vi "RTS Latest TDMS Data.vi"(6 "Number of values in file":u64, 8 "error in (no error)":errorcluster, 9 "Group":string, 10 "Channel":string, 11 "Refnum in":refnum<k34>) -> (0 "error out":errorcluster, 2 "Latest Data":dbl[](array[numeric]), 3 "Refnum out":refnum<k34>)   [LabVIEW 2016]
panel:
  in  "Read Times":i32=5
  out "number of buffers available":u32
  out "all buffers full?":bool
  out "read process finished?":bool
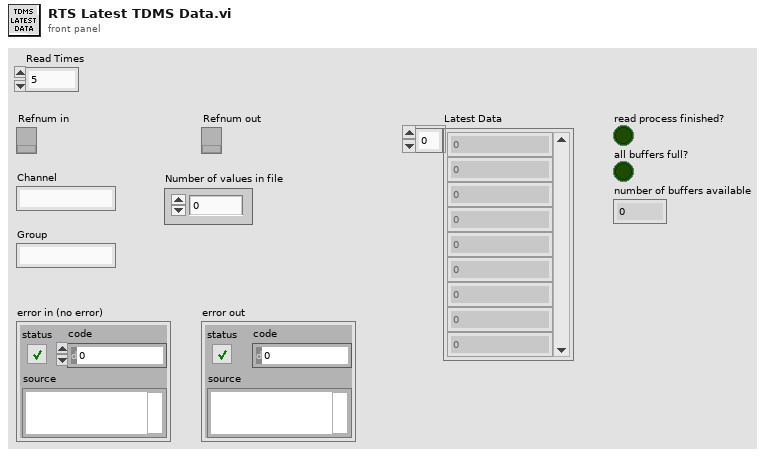
[diagram p1: front panel]
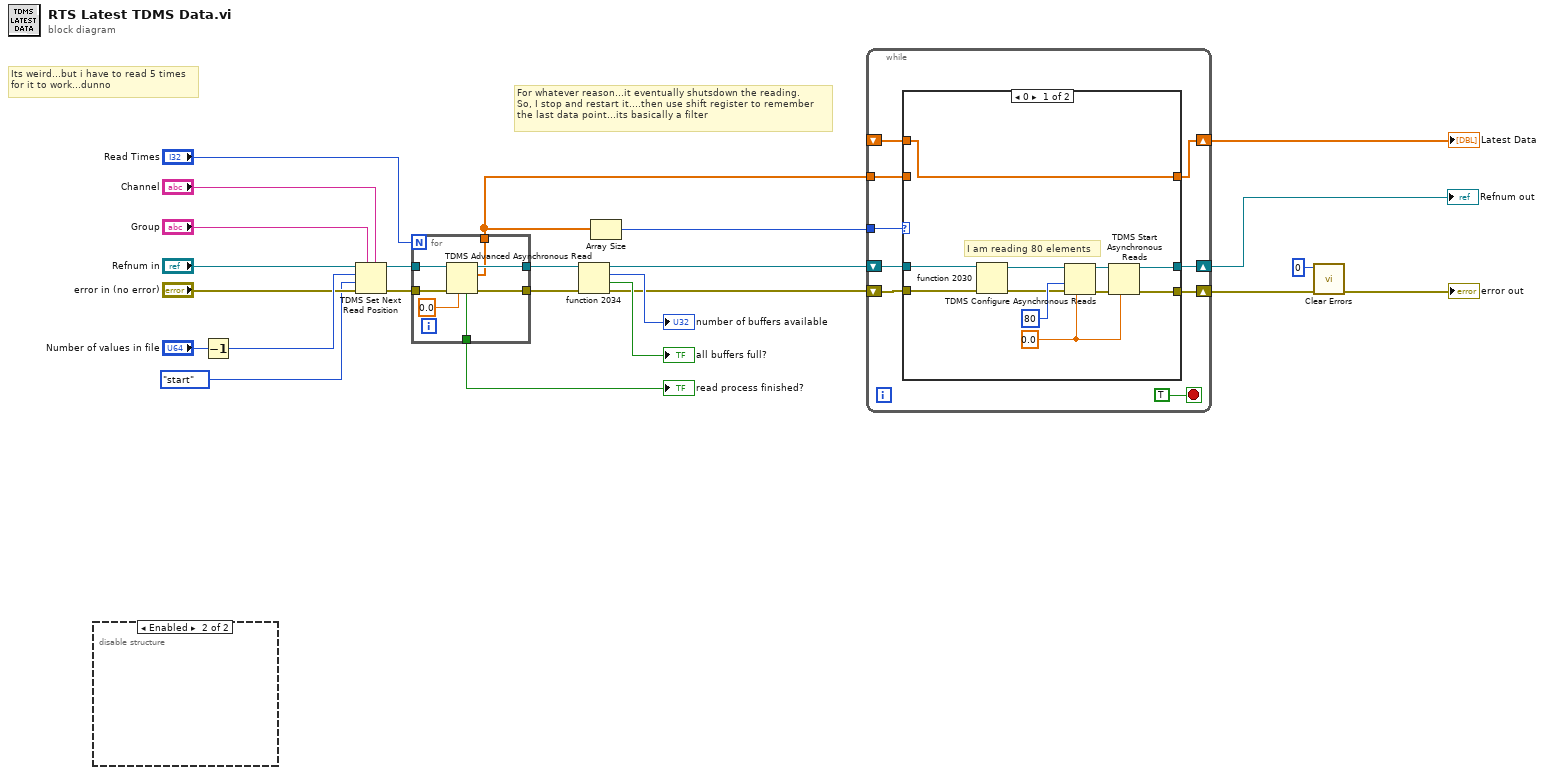
[diagram p0: block diagram]
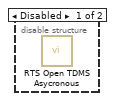
[diagram p3: hidden frame]
diagram:
  # "For whatever reason...it eventually shutsdown the reading.\nSo, I stop and restart it....then use shift register to remember\nthe last data point...its basically a filter"
  # "Its weird...but i have to read 5 times\nfor it to work...dunno"
  n1 = disable-structure shown="Enabled" {
    frame Disabled {
      n2 = call "RTS Open TDMS Asycronous.vi"() -> ()  [unwired: 10 in, 2 out]
    }
    frame Enabled {
    }
  }
  n3 = Decrement(x="Number of values in file") -> (x-1=w21:u64)
  n4 = TDMS Set Next Read Position(5:"Channel", 7:"Group", 8:"error in (no error)", 9:enum16{"start", "end"}."start" ("from (0: start)"), 10:w21, 11:"Refnum in") -> (0:w16:errorcluster, 3:w17:refnum<k34>)
  n5 = for {
    N: "Read Times" -> [_]
    tunnel: [w26] -> w5
    tunnel: w17 -> [w31]
    tunnel: [w28] -> w14
    tunnel: w16 -> [w30]
    tunnel: [w27] -> w13
    tunnel: [w25] -> w6
    n6 = TDMS Advanced Asynchronous Read(6:0.0 ("Data Type"), 8:w30, 11:w31) -> (0:w27:errorcluster, 2:w26:dbl[], 3:w28:refnum<k34>, 4:w25:bool)
  }
  "read process finished?" <- w6
  n7 = fn#2034(8:w13, 11:w14) -> (0:w9:errorcluster, 1:→"all buffers full?":bool, 2:→"number of buffers available":u32, 3:w8:refnum<k34>)
  n8 = Array Size(array=w5) -> (size(s)=w10:i32)
  n9 = while {
    tunnel: w10 -> [w38]
    tunnel: w5 -> [w35]
    shift-right: [w40] -> w3
    shift-left: w9 -> [w37]
    shift-right: [w39] -> w22
    shift-left: w8 -> [w36]
    shift-right: [w33] -> w4
    shift-left: _ -> [w32]
    stop <- TRUE stop-if-true
    n10 = case shown="0" w38 {
      tunnel: w37 -> [w51 w53]
      tunnel: w36 -> [w50 w54]
      tunnel: [w42 w54] -> w39
      tunnel: [w43 w53] -> w40
      tunnel: w35 -> [_ w52]
      tunnel: [w41 w52] -> w33
      tunnel: w32 -> [w41 _]
      frame 0 {
        w48 = 0.0 ("i16")
        # "I am reading 80 elements"
        n11 = fn#2030(8:w51, 11:w50) -> (0:w45:errorcluster, 3:w44:refnum<k34>)
        n12 = TDMS Configure Asynchronous Reads(6:w48, 8:w45, 9:u32 80 ("buffer size"), 11:w44) -> (0:w47:errorcluster, 3:w46:refnum<k34>)  [unwired: 2 in]
        n13 = TDMS Start Asynchronous Reads(6:w48, 8:w47, 11:w46) -> (0:w43:errorcluster, 3:w42:refnum<k34>)  [unwired: 1 in]
      }
      frame Default {
      }
    }
  }
  "Latest Data" <- w4
  "Refnum out" <- w22
  n14 = call <vilib>:"Clear Errors.vi"("error in (no error)"=w3, "specific error code to clear (0: all)"=0) -> ("error out"=→"error out":errorcluster)  [unwired: 4 in, 1 out]
